vi "Read YOLO INI.vi"(0 "Path to INI":path) -> (11 "OUTPUT_NAME":string, 12 "ANCHORS":sgl[](array[numeric]), 13 "INPUT_NAME":string, 14 "IMAGE_H":i32, 15 "IMAGE_W":i32, 16 "GRID_H":i32, 17 "GRID_W":i32, 18 "BOXES":i32, 19 "CLASSES":i32)   [LabVIEW 2016]
uses:
  <vilib>/Utility/config.llb/Read Key (I32).vi
  <vilib>/Utility/config.llb/Read Key (String).vi
  <vilib>/Utility/config.llb/NI_LVConfig.lvlib
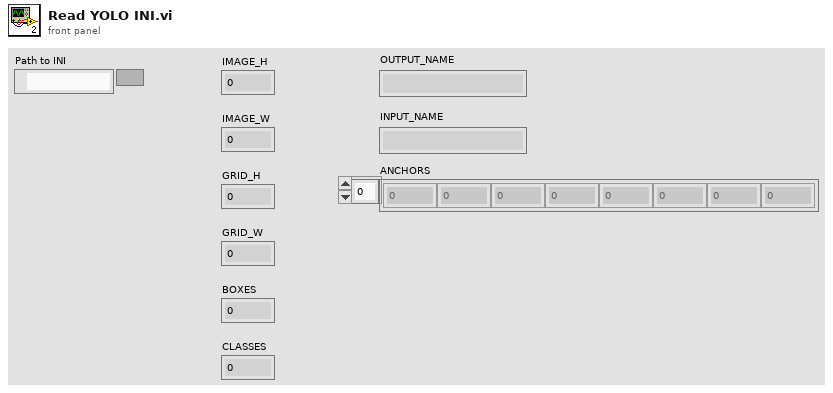
[diagram p1: front panel]
types:
  T1 = typedef "NI_LVConfig.lvlib/Config Data RefNum.ctl" = refnum<k1>
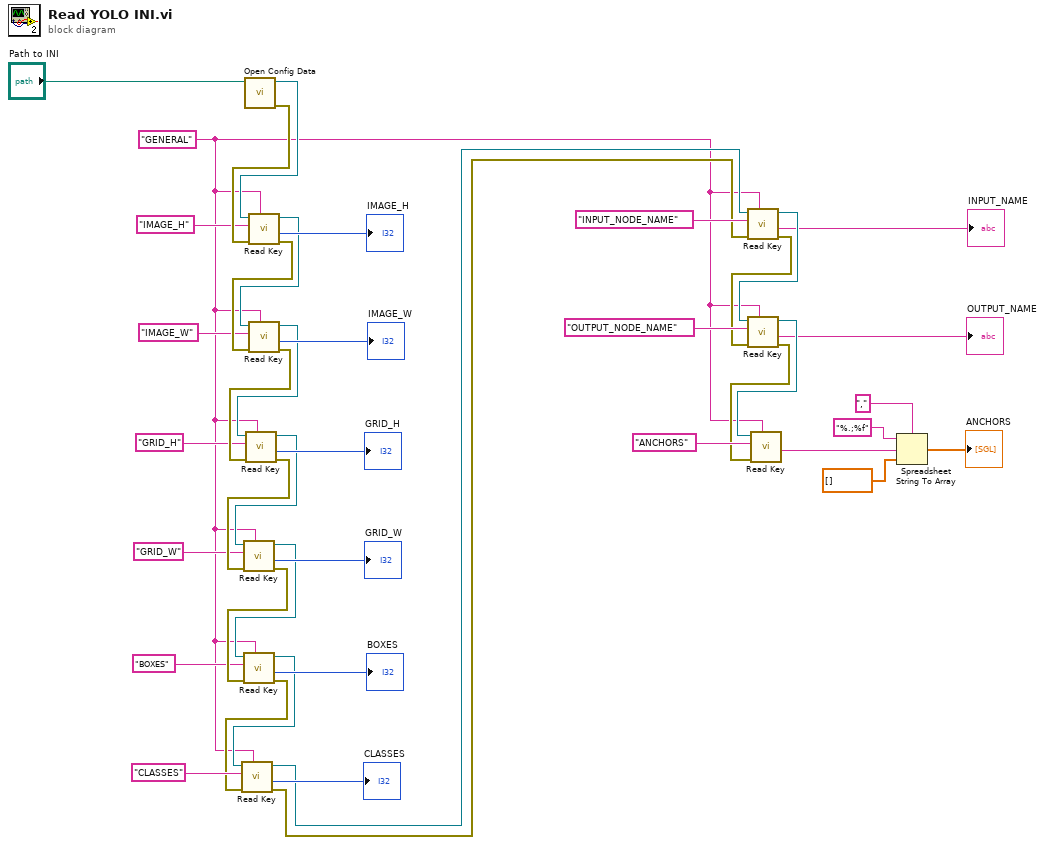
[diagram p0: block diagram]
diagram:
  w1 = "GENERAL" ("section")
  n1 = call <vilib>:"Open Config Data.vi"("configuration file path"="Path to INI") -> ("error out"=w13:errorcluster, "refnum"=w14:T1)  [unwired: 8 in, 1 out]
  n2 = call-poly <vilib>:"Read Key.vi"("section"=w1, "error in (no error)"=w13, "key"="IMAGE_H", "refnum"=w14) -> ("error out"=w16:errorcluster, "value"=→"IMAGE_H":i32, "refnum out"=w17:T1)  [unwired: 4 in, 1 out]
  n3 = call-poly <vilib>:"Read Key.vi"("section"=w1, "error in (no error)"=w16, "key"="IMAGE_W", "refnum"=w17) -> ("error out"=w21:errorcluster, "value"=→"IMAGE_W":i32, "refnum out"=w20:T1)  [unwired: 4 in, 1 out]
  n4 = call-poly <vilib>:"Read Key.vi"("section"=w1, "error in (no error)"=w21, "key"="GRID_H", "refnum"=w20) -> ("error out"=w23:errorcluster, "value"=→"GRID_H":i32, "refnum out"=w22:T1)  [unwired: 4 in, 1 out]
  n5 = call-poly <vilib>:"Read Key.vi"("section"=w1, "error in (no error)"=w23, "key"="GRID_W", "refnum"=w22) -> ("error out"=w28:errorcluster, "value"=→"GRID_W":i32, "refnum out"=w29:T1)  [unwired: 4 in, 1 out]
  n6 = call-poly <vilib>:"Read Key.vi"("section"=w1, "error in (no error)"=w28, "key"="BOXES", "refnum"=w29) -> ("error out"=w24:errorcluster, "value"=→"BOXES":i32, "refnum out"=w25:T1)  [unwired: 4 in, 1 out]
  n7 = call-poly <vilib>:"Read Key.vi"("section"=w1, "error in (no error)"=w24, "key"="CLASSES", "refnum"=w25) -> ("error out"=w6:errorcluster, "value"=→"CLASSES":i32, "refnum out"=w7:T1)  [unwired: 4 in, 1 out]
  n8 = call-poly <vilib>:"Read Key.vi"("section"=w1, "error in (no error)"=w6, "key"="INPUT_NODE_NAME", "refnum"=w7) -> ("error out"=w9:errorcluster, "value"=→"INPUT_NAME":string, "refnum out"=w8:T1)  [unwired: 4 in, 1 out]
  n9 = call-poly <vilib>:"Read Key.vi"("section"=w1, "error in (no error)"=w9, "key"="OUTPUT_NODE_NAME", "refnum"=w8) -> ("error out"=w4:errorcluster, "value"=→"OUTPUT_NAME":string, "refnum out"=w5:T1)  [unwired: 4 in, 1 out]
  n10 = call-poly <vilib>:"Read Key.vi"("section"=w1, "error in (no error)"=w4, "key"="ANCHORS", "refnum"=w5) -> ("value"=w36:string)  [unwired: 4 in, 3 out]
  n11 = Spreadsheet String To Array(delimiter (Tab)=",", format string="%.;%f", spreadsheet string=w36, array type (2D Dbl)=sgl[] []) -> (array=→"ANCHORS":sgl[])
